vi "APS get vao param ex.vi"(8 "error in (no error)":errorcluster caption="错误输入（无错误）", 9 "VaoData":T1, 10 "Table_No":i32, 11 "Board_ID":i32) -> (0 "error out":errorcluster caption="错误输出", 1 "VaoData out":T1, 3 "function return":i32)   [LabVIEW 2011, in "APS168.lvlib"]
doc: "I32 FNTYPE APS_get_vao_param_ex( I32 Board_ID, I32 Table_No, VAO_DATA* VaoData );"
uses:
  APS168.lvlib
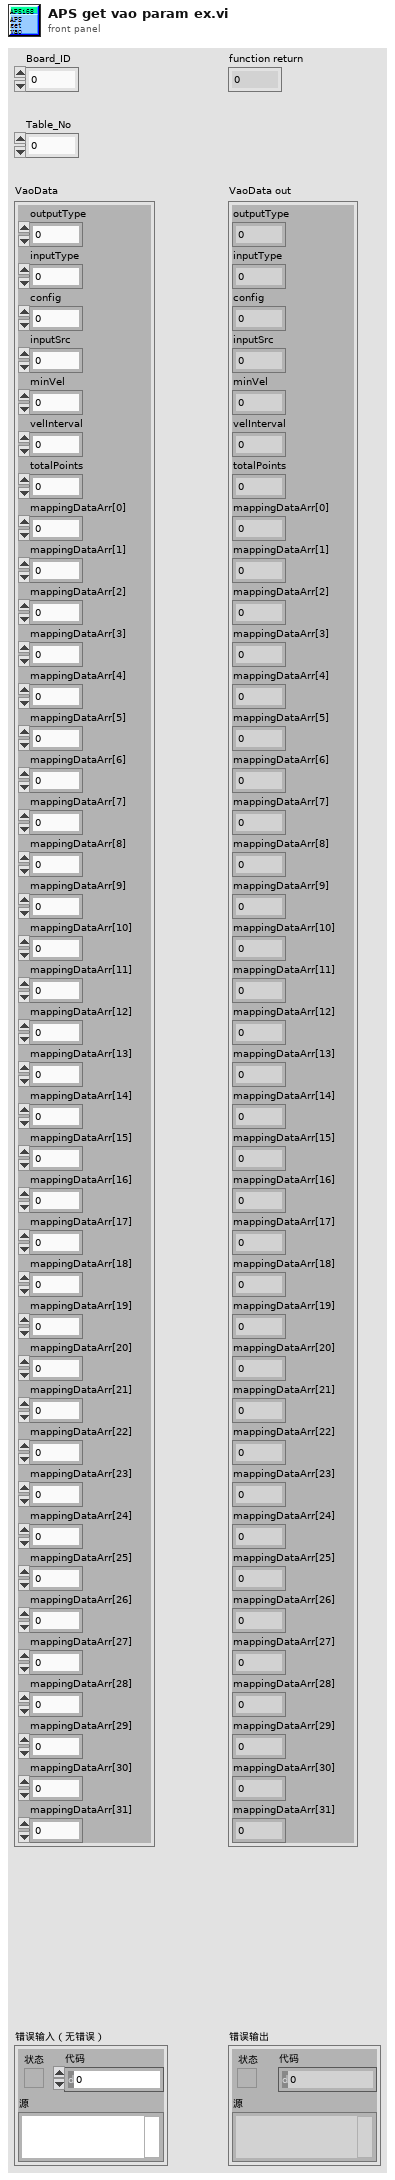
[diagram p1: front panel]
types:
  T1 = cluster{"outputType":i32, "inputType":i32, "config":i32, "inputSrc":i32, "minVel":i32, "velInterval":i32, "totalPoints":i32, "mappingDataArr[0]":i32, "mappingDataArr[1]":i32, "mappingDataArr[2]":i32, "mappingDataArr[3]":i32, "mappingDataArr[4]":i32, "mappingDataArr[5]":i32, "mappingDataArr[6]":i32, "mappingDataArr[7]":i32, "mappingDataArr[8]":i32, "mappingDataArr[9]":i32, "mappingDataArr[10]":i32, "mappingDataArr[11]":i32, "mappingDataArr[12]":i32, "mappingDataArr[13]":i32, "mappingDataArr[14]":i32, "mappingDataArr[15]":i32, "mappingDataArr[16]":i32, "mappingDataArr[17]":i32, "mappingDataArr[18]":i32, "mappingDataArr[19]":i32, "mappingDataArr[20]":i32, "mappingDataArr[21]":i32, "mappingDataArr[22]":i32, "mappingDataArr[23]":i32, "mappingDataArr[24]":i32, "mappingDataArr[25]":i32, "mappingDataArr[26]":i32, "mappingDataArr[27]":i32, "mappingDataArr[28]":i32, "mappingDataArr[29]":i32, "mappingDataArr[30]":i32, "mappingDataArr[31]":i32}
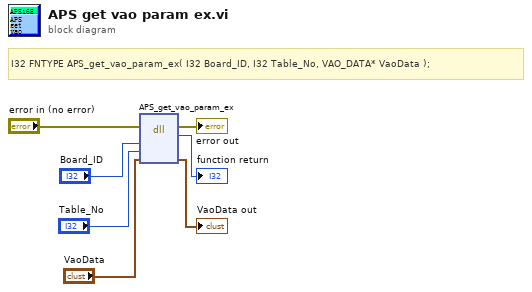
[diagram p0: block diagram]
diagram:
  # "I32 FNTYPE APS_get_vao_param_ex( I32 Board_ID, I32 Table_No, VAO_DATA* VaoData );"
  n1 = dll-call lib="PTH1Labs E软件ADLINK 204CAPS_1_7_1_LIB line 连续运动204APS168.*" fn="APS_get_vao_param_ex"(error in="error in (no error)", "Board_ID"="Board_ID", "Table_No"="Table_No", "VaoData"="VaoData") -> (error out=→"error out":errorcluster, →"function return":i32, "VaoData"=→"VaoData out":T1)  [unwired: 4 in, 1 out]
